vi "GLdrv_FILE_LIST_FORM_FILT.vi"(0 "Connection ID":T1, 5 "Format":enum16{"SHORT", "LONG"}(ring), 7 "Filter":string, 11 "error in (no error)":errorcluster, 13 "Query(f)":bool) -> (4 "Connection ID Out":T1, 6 "Format out":enum16{"SHORT", "LONG"}(ring), 8 "Filter out":string, 15 "error out":errorcluster)   [LabVIEW 2017, in "GL860_Driver.lvlib"]
doc: "FORM：　ファイル表示のフォーマットを設定します\nSHORT：　ファイル名のみ\nLONG：　ファイル名+日付+サイズ+属性\nFILT: 表示するファイルを拡張子によって制限します\n<拡張子>：　“.***”ドット付き4文字\nフィルタで設定した拡張子ファイルのみ表示\nOFF：　すべてのファイルを表示する\n\n:FILE:LIST:FORM SHORT時のレスポンス例\n（ルート時：接続されているデバイスを表示する）\n:FILE:LIST “MEM\\”,”SD\\”\n（ルート以外の時）\n:FILE:LIST “FOLDER\\”,”FOLDER2\\”,“050101-\n010101.GBD”,”050502-010101.GBD”\n:FILE:LIST:FORM LONG時のレスポンス例\n（ルート時：接続されているデバイスを表示する） <デバイス> <空き容\n量> <属性>\n:FILE:LIST “MEM\\ 123456 d--”,”SD\\ 123456 d--”\n（ルート以外の時） <ファイル/フォルダ> <作成日> <属性>\n:FILE:LIST “FOLDER\\ 2012/01/01 12:34:56 dw-\n”,”FOLDER2\\ 2012/01/01 12:34:57 dw-”,“120101-010101.GBD\n2012/01/01 12:34:56 -w-”,”120502-123456.GBD 2012/05/02\n12:34:56 -w-”\n\n属性　説明\ndw-　書き込み可能なディレクトリ（フォルダ）\n-w-　書き込み可能なファイル"
uses:
  GL860_Driver.lvlib
  ConnectionID.ctl
  GLdrv_RW.ctl
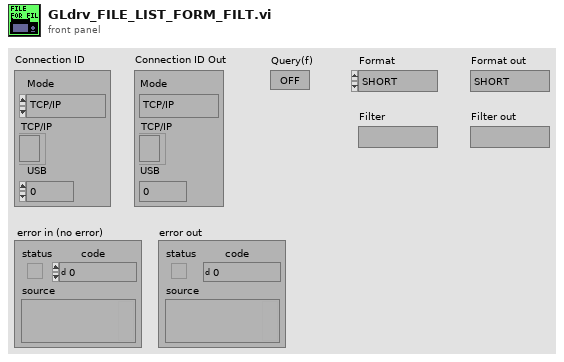
[diagram p1: front panel]
types:
  T1 = typedef "ConnectionID.ctl" = cluster{"Mode":enum16{"TCP/IP", "USB"}, "TCP/IP":refnum<k5>, "USB":i32}
  T2 = typedef "GLdrv_RW.ctl" = enum16{"Auto", "Read", "Write", "Buffer"}
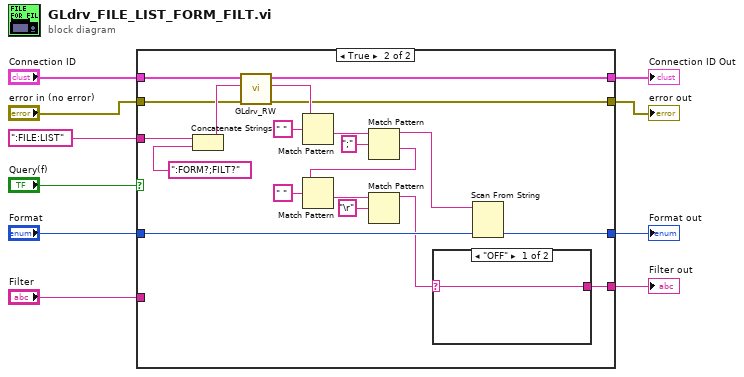
[diagram p0: block diagram]
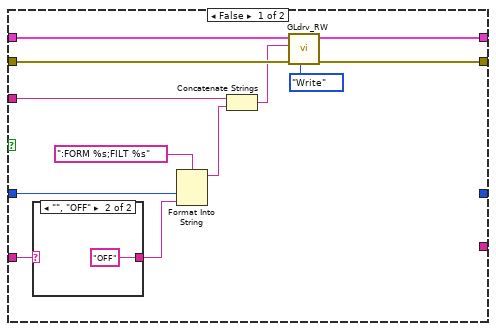
[diagram p2: hidden frame]
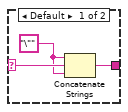
[diagram p3: hidden frame]
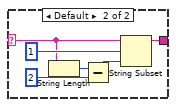
[diagram p4: hidden frame]
diagram:
  n1 = case shown="TRUE" "Query(f)" {
    tunnel: ":FILE:LIST" ("Command") -> [w22 w45]
    tunnel: [w18 w39] -> w10
    tunnel: [w20 w43] -> w9
    tunnel: "Connection ID" -> [w21 w44]
    tunnel: "error in (no error)" -> [w19 w40]
    tunnel: "Format" -> [w14 w30]
    tunnel: "Filter" -> [w12 _]
    tunnel: [_ w29] -> w2
    tunnel: [_ w28] -> w1
    frame False {
      n2 = case shown="\"\", \"OFF\"" w12 {
        selector: w12 -> [w25 _]
        tunnel: [w24 "OFF"] -> w11
        frame Default {
          w23 = "\"" ("string")
          n3 = Concatenate Strings(w23, w25, w23) -> (w24:string)
        }
        frame "", "OFF" {
        }
      }
      n4 = Format Into String(format string=":FORM %s;FILT %s" ("string"), w14, w11) -> (resulting string=w15:string)  [unwired: 2 in, 1 out]
      n5 = Concatenate Strings(w22, w15) -> (w17:string)
      n6 = call "GLdrv_RW.vi"("Mode(read)"=GLdrv_RW."Write", "error in (no error)"=w19, "data in"=w17, "Connection ID"=w21) -> ("error out"=w18:errorcluster, "Connection ID Out"=w20:T1)  [unwired: 3 in, 3 out]
    }
    frame True {
      n7 = Concatenate Strings(w45, ":FORM?;FILT?" ("string")) -> (w42:string)
      n8 = call "GLdrv_RW.vi"("error in (no error)"=w40, "data in"=w42, "Connection ID"=w44) -> ("error out"=w39:errorcluster, "data out"=w41:string, "Connection ID Out"=w43:T1)  [unwired: 4 in, 2 out]
      n9 = Match Pattern(string=w41, regular expression=" " ("search string/char (-)")) -> (after substring=w36:string)  [unwired: 4 out]
      n10 = Match Pattern(string=w36, regular expression=";" ("search string/char (-)")) -> (before substring=w31:string, after substring=w32:string)  [unwired: 3 out]
      n11 = Match Pattern(string=w32, regular expression=" " ("search string/char (-)")) -> (after substring=w35:string)  [unwired: 4 out]
      n12 = Match Pattern(string=w35, regular expression="\r" ("search string/char (-)")) -> (before substring=w27:string)  [unwired: 4 out]
      n13 = case shown="\"OFF\"" w27 {
        selector: w27 -> [w47 w48]
        tunnel: [w47 w49] -> w28
        frame "OFF" {
        }
        frame Default {
          n14 = String Length(string=w48) -> (length=w51:i32)
          n15 = Subtract(x=w51, y=2) -> (x-y=w52:i32)
          n16 = String Subset(string=w48, offset (0)=1, length (rest)=w52) -> (substring=w49:string)
        }
      }
      n17 = Scan From String(input string=w31, default 1=w30) -> (output 1=w29:enum16{"SHORT", "LONG"})  [unwired: 3 in, 3 out]
    }
  }
  "Connection ID Out" <- w9
  "error out" <- w10
  "Format out" <- w2
  "Filter out" <- w1
